vi "DialogCreateInterface.vi"(0 "ClassWriter in":refnum<class "ClassWriter.lvclass">, 1 "ProjectItem Refnum":refnum<vi>, 5 "error in (no error)":errorcluster) -> (14 "ClassWriter out":refnum<class "ClassWriter.lvclass">, 15 "Cancelled":bool, 16 "CreateInterfaceData":T1, 19 "error out":errorcluster)   [LabVIEW 2020, in "ClassWriter.lvclass"]
uses:
  ClassWriter.lvclass
  CreateInterfaceData.ctl
  InterfaceMethodsToCreate.ctl
  Common/CommonVIs/CommonVIs_AttributeType.ctl
  Common/CommonVIs/CommonVIs_AttributeDataType.ctl
  Common/String/GDSString_AccessScopeModifierType.ctl
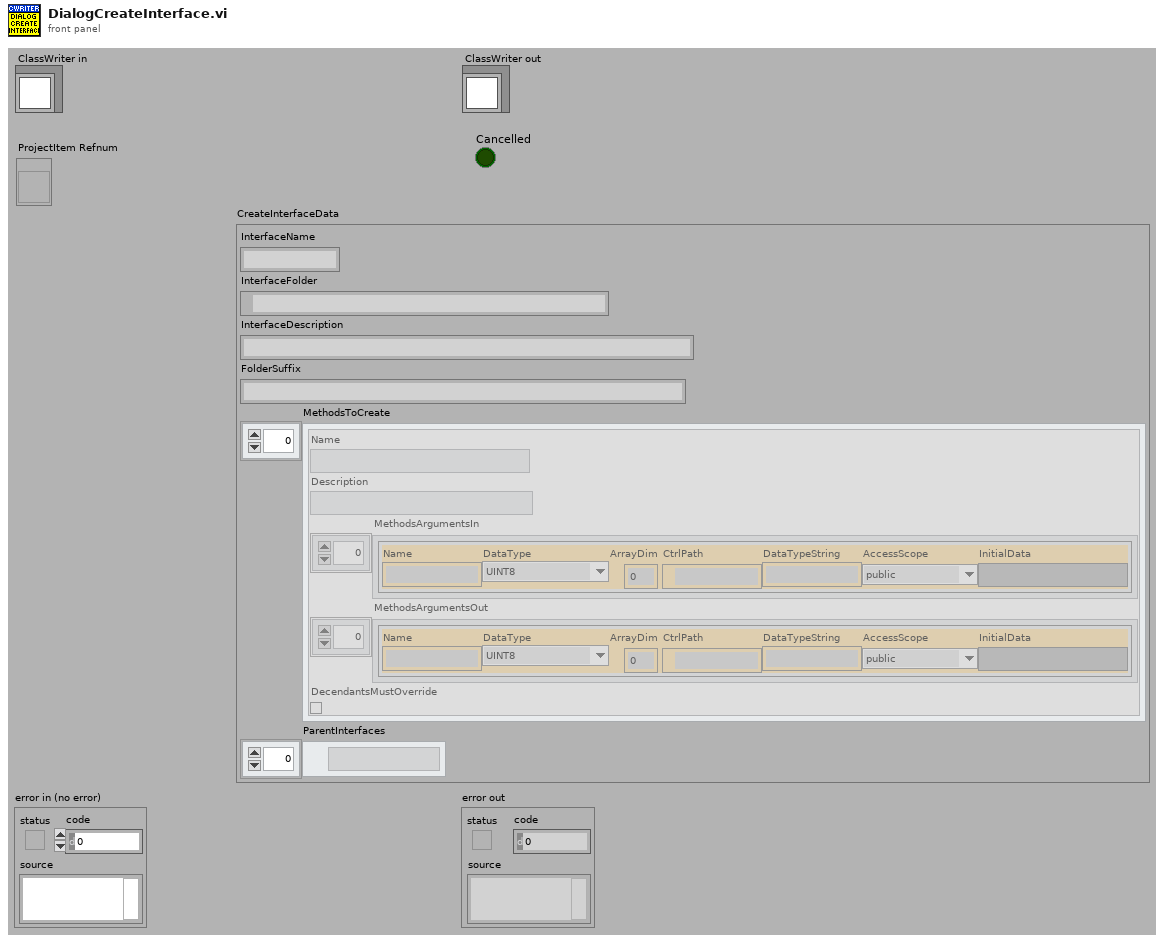
[diagram p1: front panel]
types:
  T1 = typedef "ClassWriter.lvclass/CreateInterfaceData.ctl" = cluster{"InterfaceName":string, "InterfaceFolder":path, "InterfaceDescription":string, "FolderSuffix":string, "MethodsToCreate":T2[], "ParentInterfaces":path[]}
  T2 = typedef "ClassWriter.lvclass/InterfaceMethodsToCreate.ctl" = cluster{"Name":string, "Description":string, "MethodsArgumentsIn":T3[], "MethodsArgumentsOut":T3[], "DecendantsMustOverride":bool}
  T3 = typedef "CommonVIs_AttributeType.ctl" = cluster{"Name":string, "DataType":T4, "ArrayDim":i32, "CtrlPath":path, "DataTypeString":string, "AccessScope":T5, "InitialData":variant}
  T4 = typedef "CommonVIs_AttributeDataType.ctl" = enum16{"UINT8", "INT8", "UINT16", "INT16", "UINT32", "INT32", "UINT64", "INT64", "SGL", "DBL", "EXT", "CSG", "CDB", "CXT", "TimeStamp", "STRING", "PATH", "BOOL", "ENUM", "RefNum", "VIRefNum", "LabVIEW Class", "Cluster", "Variant", "TypeDef", "Waveform", "LabVIEW Object", "Other", "void", "Set", "Map"}
  T5 = typedef "GDSString_AccessScopeModifierType.ctl" = enum16{"public", "private", "protected", "internal"}
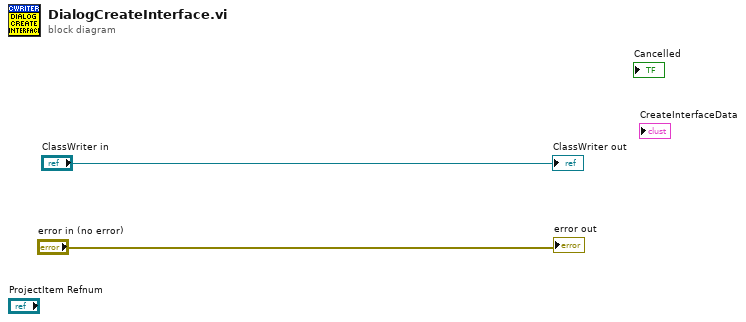
[diagram p0: block diagram]
diagram:
  "error out" <- "error in (no error)"
  "ClassWriter out" <- "ClassWriter in"
